vi "oax_gsTimebase Plot.vi"() -> ()   [LabVIEW 2017]
doc: "This is Order Analysis Toolkit demo VI."
uses:
  <vilib>/addons/Sound and Vibration/Order Analysis/Tach Process/SoundVib_TachProcess.lvlib
  <vilib>/addons/Sound and Vibration/Order Analysis/Resample Order Tracking/SoundVib_OrderTracking.lvlib
  <vilib>/Waveform/WDTOps.llb/WDT Waveform Duration DBL.vi
  <vilib>/addons/Sound and Vibration/Order Analysis/Data Presentation/SoundVib_MCMDisplay.lvlib
  <vilib>/addons/Sound and Vibration/Order Analysis/Data Presentation/SVX Orbit and Timebase Plot (Unfiltered).vi
  <vilib>/addons/Sound and Vibration/Order Analysis/Data Presentation/SubVIs/OAT MCM Channel Property.ctl
  <vilib>/addons/Sound and Vibration/Order Analysis/Data Presentation/SVX Orbit and Timebase Plot (Filtered) (N Ch - 1 Order).vi
  <vilib>/addons/_XControls/Timebase Plot/SVX Timebase.xctl
panel:
  in  "samples/rev wanted":i32=64
  in  "order to display":dbl=1.0 min=0.0 format="%.2f"
  in  "plot type":u16(ring) items=["unfiltered plot", "filtered plot"]
  in  "timebase plot display revolutions":cluster{"duration [rev]":dbl}={"duration [rev]"=8.0} {"duration [rev]" format="%.2f"}
  out "Timebase plot":T1(xcontrol) caption="Y axis"
  in  "STOP":bool
  in  "Select Data":i32(listbox)
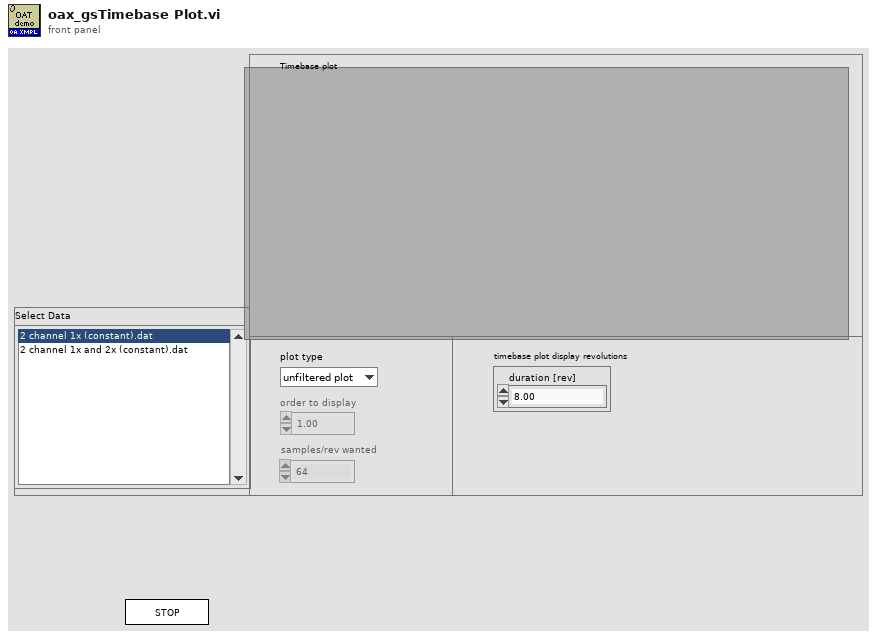
[diagram p1: front panel]
types:
  T1 = cluster{"X":dbl[], "Y":dbl[], "reference":dbl[], "plot type":enum16{"Filtered Plot", "Unfiltered Plot"}, "attribute":variant}[][]
  T2 = typedef "OAT MCM Channel Property.ctl" = cluster{"direction":u16, "probe angle [deg]":u16, "pair":u16}
  T3 = cluster{"unwrap phase? (T)":bool, "unit in degree? (F)":bool, "unwrap phase? (T) 2":bool}
  T4 = typedef "SoundVib_TachProcess.lvlib/speed profile.ctl" = cluster{"time [s]":dbl[], "speed [RPM]":dbl[]}
  T5 = typedef "svc_Resampled Channel Info.ctl" = cluster{"channel name":string, "description":string, " channel info":T6}
  T6 = typedef "svc_Channel Info.ctl" = cluster{"sensor sensitivity":dbl, "engineering units":T7, "dB reference":dbl, "custom label":string, "weighting filter":T8, "pregain":dbl}
  T7 = typedef "svc_Engineering Units Text Ring.ctl" = u16
  T8 = typedef "svc_Weighting Filter Text Ring.ctl" = u16
  T9 = typedef "OAT Position Info.ctl" = cluster{"positions [s]":dbl[], "samples/rev":dbl}
  T10 = cluster{"probe x":dbl[], "probe y":dbl[], "reference":dbl[], "plot type":enum16{"Filtered Plot", "Unfiltered Plot"}, "attribute":variant}[][]
  T11 = cluster{"time/rev/rpm":dbl[], "magnitude":dbl[]}[][]
  T12 = typedef "svc_Spectrum Info.ctl" = cluster{"channel name":string, "description":string, "x-axis units":T13, "spectral info":cluster{"spectrum type":T14, "linear/dB":enum16{"linear", "dB"}, "window":u16, "window size":i32, "FFT size":i32}, "engineering units":T7, "custom label":string, "dB reference [EU]":dbl, "peak units":enum16{"rms", "peak", "peak-peak"}, "weighting filter":T8, "spectral density?":bool, "unit label":string, "spectrum skewed?":bool, "complimentary spectrum units":T15}
  T13 = typedef "svc_X-Axis Units.ctl" = u16
  T14 = typedef "svc_Spectrum Type.ctl" = enum16{"FFT Spectrum [complex]", "Amplitude [Magnitude]", "Power [Magnitude^2]", "Cross Spectrum [complex]", "Frequency Response [Complex]"}
  T15 = typedef "svc_Complimentary Spectrum Units.ctl" = enum16{"none", "radians", "degrees", "cycles", "imaginary"}
  T16 = cluster{"time/rev/rpm":dbl[], "magnitude":dbl[]}[]
  T17 = cluster{"pulse / rev":i32, "threshold (auto)":dbl, "slope (Rising)":u16}
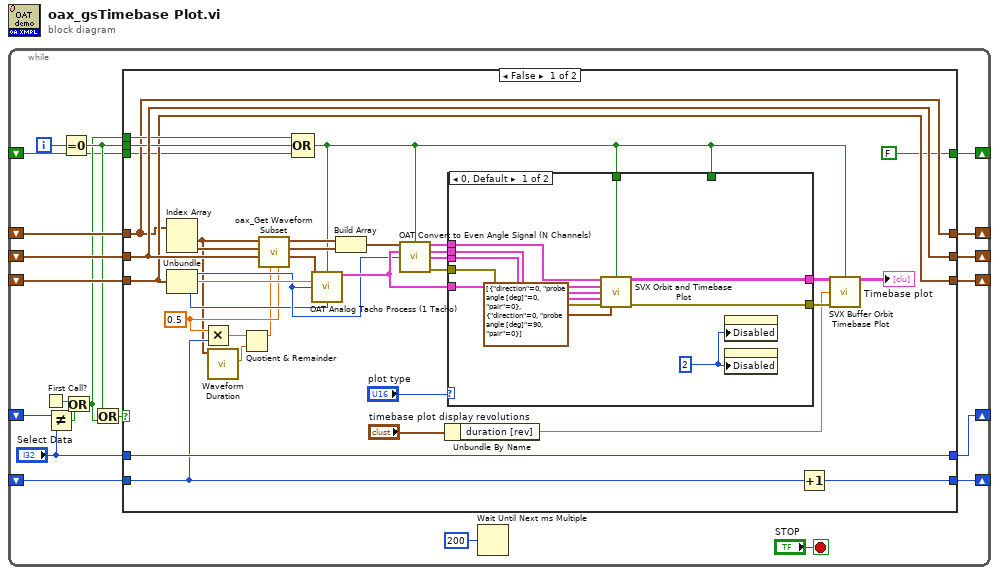
[diagram p0: block diagram]
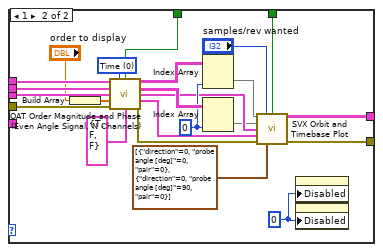
[diagram p2: hidden frame]
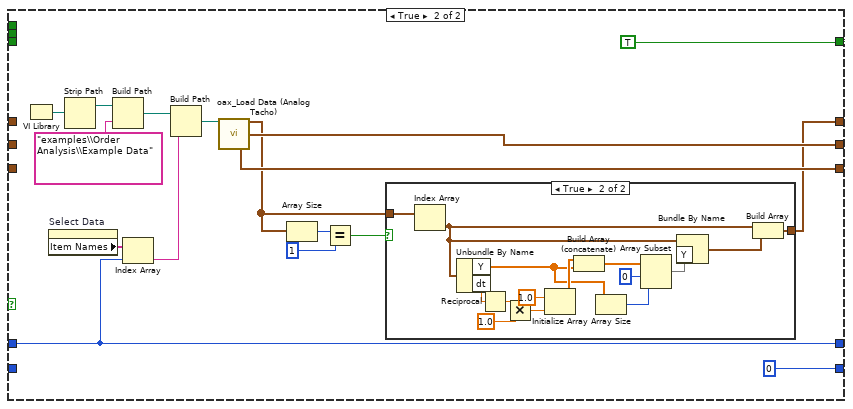
[diagram p3: hidden frame]
diagram:
  n1 = while {
    shift-right: [w17] -> _
    shift-left: _ -> [w18]
    shift-right: [w15] -> _
    shift-left: _ -> [w21]
    shift-right: [w14] -> _
    shift-left: _ -> [w19]
    shift-right: [w13] -> _
    shift-left: _ -> [w12]
    shift-right: [w3] -> _
    shift-left: _ -> [w4]
    shift-right: [w2] -> _
    shift-left: _ -> [w1]
    i -> [w11]
    stop <- "STOP" stop-if-true
    n2 = First Call?() -> (First Call?: T/F=w7:bool)
    n3 = Not Equal?(x=w18, y="Select Data") -> (x != y?=w6:bool)
    n4 = Equal To 0?(x=w11) -> (x = 0?=w10:bool)
    n5 = Or(x=w7, y=w6) -> (x .or. y?=w5:bool)
    n6 = Or(x=w10, y=w5) -> (x .or. y?=w9:bool)
    n7 = case shown="False" w9 {
      tunnel: w21 -> [w36 _]
      tunnel: w19 -> [w54 _]
      tunnel: [w55 w105] -> w17
      tunnel: "Select Data" -> [w55 w105]
      tunnel: [w36 w90] -> w15
      tunnel: [w54 w103] -> w14
      tunnel: [w47 w102] -> w13
      tunnel: w12 -> [w47 _]
      tunnel: w5 -> [w51 _]
      tunnel: w10 -> [w50 _]
      tunnel: w4 -> [w41 _]
      tunnel: [w43 0] -> w3
      tunnel: [FALSE TRUE] -> w2
      tunnel: w1 -> [w35 _]
      frame False {
        w42 = 0.5 ("y")
        n8 = Index Array(array=w36) -> (element #1=w40:waveform(dbl), element #2=w48:waveform(dbl))  [unwired: 2 in]
        n9 = Unbundle(w47) -> ("pulse / rev"=w45:i32, "threshold (auto)"=w46:dbl, "slope (Rising)"=w44:u16)
        n10 = Multiply(x=w42, y=w41) -> (x*y=w38:dbl)
        n11 = call-poly <vilib>:"Waveform Duration.vi"("waveform in"=w40) -> ("duration"=w39:dbl)  [unwired: 8 in, 2 out]
        n12 = Quotient & Remainder(x=w38, y=w39) -> (x-y*floor(x/y)=w37:dbl)  [unwired: 1 out]
        n13 = call <vilib>:"oax_Get Waveform Subset.vi"("duration"=w42, "start index"=w37, "Tach Signal"=w54, "Vibration Signal Y"=w48, "Vibration Signal X"=w40) -> ("Tach Signal out"=w52:waveform(dbl), "Vibration Signal Y out"=w53:waveform(dbl), "Vibration Signal X out"=w49:waveform(dbl))  [unwired: 3 in, 1 out]
        n14 = Compound Arithmetic op=OR(w51, w50, w35) -> (w26:bool)
        n15 = call <vilib>:"OAT Analog Tacho Process (1 Tacho).vi"("analog tacho signal"=w52, "reset? (F)"=w26, "threshold (auto)"=w46, "pulse/revolution (1)"=w45, "slope (Rising)"=w44) -> ("speed profile"=w56:T4)  [unwired: 6 in, 4 out]
        n16 = Build Array(w49, w53) -> (w33:waveform(dbl)[])
        n17 = call <vilib>:"OAT Convert to Even Angle Signal (N Channels).vi"("scaled signals [EU]"=w33, "reset? (F)"=w26, "speed profile"=w56, "pulse/revolution (1)"=w45) -> ("even-angle signals"=w32:cluster{"r0":dbl, "dr":dbl, "Y":dbl[]}[], "even-angle channel info"=w30:T5[], "even-angle position info"=w31:T9, "error out"=w29:errorcluster)  [unwired: 7 in, 1 out]
        n18 = Unbundle By Name("timebase plot display revolutions") -> ("duration [rev]"=w22:dbl)
        n19 = case shown="0, Default" "plot type" {
          tunnel: w32 -> [w61 w89]
          tunnel: w56 -> [w65 _]
          tunnel: w31 -> [w64 w87]
          tunnel: [w66 w68] -> w27
          tunnel: w30 -> [w60 w88]
          tunnel: w29 -> [w59 w86]
          tunnel: w26 -> [w63 w83]
          tunnel: w26 -> [_ w77]
          tunnel: [w57 w67] -> w24
          frame 0, Default {
            w62 = u8 2 ("Disabled")
            n20 = call-poly <vilib>:"SVX Orbit and Timebase Plot.vi"("even-angle signals"=w61, "reset? (F)"=w63, "even-angle channel info"=w60, "even-angle position info"=w64, "speed profile"=w65, "error in (no error)"=w59, "channel properties"=T2[] [{"direction"=0, "probe angle [deg]"=0, "pair"=0}, {"direction"=0, "probe angle [deg]"=90, "pair"=0}]) -> ("orbit/timebase plot"=w66:T10, "error out"=w57:errorcluster)  [unwired: 5 in, 2 out]
            n21 = property on="order to display" class="DigNum (strict)"("Disabled"=w62) -> ()  [unwired: 2 in, 2 out]
            n22 = property on="samples/rev wanted" class="DigNum (strict)"("Disabled"=w62) -> ()  [unwired: 2 in, 2 out]
          }
          frame 1 {
            w78 = u8 0 ("Disabled")
            w79 = u16 0 items=["Time", "Revolution", "RPM"] ("X axis selection")
            w80 = 0 ("disabled index (col)")
            n23 = Build Array("order to display") -> (w82:dbl[])
            n24 = call <vilib>:"OAT Order Magnitude and Phase (Even Angle Signal, N Channels).vi"("even-angle signals"=w89, "x-axis selection"=w79, "reset? (F)"=w83, "even-angle channel info"=w88, "even-angle position info"=w87, "orders to compute (1.0)"=w82, "error in (no error)"=w86, "view"=T3 {"unwrap phase? (T)"=TRUE, "unit in degree? (F)"=FALSE, "unwrap phase? (T) 2"=FALSE} ("phase setting")) -> ("magnitudes [RMS]"=w85:T11, "phases [phase lag]"=w84:cluster{"time/rev/rpm":dbl[], "phase":dbl[]}[][], "magnitude/phase position info"=w73:T9, "magnitudes info"=w70:T12[], "error out"=w81:errorcluster)  [unwired: 2 in, 1 out]
            n25 = Index Array(array=w85, index (col)=w80) -> (element=w74:T16)  [unwired: 1 in]
            n26 = Index Array(array=w84, index (col)=w80) -> (element=w72:cluster{"time/rev/rpm":dbl[], "phase":dbl[]}[])  [unwired: 1 in]
            n27 = call-poly <vilib>:"SVX Orbit and Timebase Plot.vi"("magnitudes [RMS]"=w74, "samples/rev wanted"="samples/rev wanted", "reset? (F)"=w77, "phases [phase lag]"=w72, "magnitude/phase position info"=w73, "magnitudes info"=w70, "error in (no error)"=w81, "channel properties"=T2[] [{"direction"=0, "probe angle [deg]"=0, "pair"=0}, {"direction"=0, "probe angle [deg]"=90, "pair"=0}]) -> ("orbit/timebase plot"=w68:T10, "error out"=w67:errorcluster)  [unwired: 4 in, 2 out]
            n28 = property on="order to display" class="DigNum (strict)"("Disabled"=w78) -> ()  [unwired: 2 in, 2 out]
            n29 = property on="samples/rev wanted" class="DigNum (strict)"("Disabled"=w78) -> ()  [unwired: 2 in, 2 out]
          }
        }
        n30 = Increment(x=w41) -> (x+1=w43:i32)
        n31 = call <vilib>:"SVX Buffer Orbit Timebase Plot.vi"("orbit/timebase plot in"=w27, "reset? (F)"=w26, "buffer size (rev)"=w22, "error in (no error)"=w24) -> ("orbit/timebase plot out"=→"Timebase plot":T10)  [unwired: 10 in, 1 out]
      }
      frame True {
        n32 = VI Library() -> (path=w98:path)
        n33 = property on="Select Data" class="LstBox (strict)"() -> ("Item Names"=w106:string[])  [unwired: 2 in, 2 out]
        n34 = Strip Path(path=w98) -> (stripped path=w97:path)  [unwired: 1 out]
        n35 = Build Path(base path=w97, name or relative path="examples\\Order Analysis\\Example Data") -> (appended path=w101:path)
        n36 = Index Array(array=w106, index=w105) -> (element=w100:string)
        n37 = Build Path(base path=w101, name or relative path=w100) -> (appended path=w99:path)
        n38 = call <vilib>:"oax_Load Data (Analog Tacho).vi"("Data Path In"=w99) -> ("vibration data"=w91:waveform(dbl)[], "analog tacho signal"=w103:waveform(dbl), "tacho info"=w102:T17)  [unwired: 8 in, 4 out]
        n39 = Array Size(array=w91) -> (size(s)=w94:i32)
        n40 = Equal?(x=w94, y=1) -> (x = y?=w92:bool)
        n41 = case shown="True" w92 {
          tunnel: w91 -> [w107 w122]
          tunnel: [w107 w121] -> w90
          frame False {
          }
          frame True {
            n42 = Index Array(array=w122) -> (element=w120:waveform(dbl))  [unwired: 1 in]
            n43 = Unbundle By Name(w120) -> ("Y"=w109:dbl[], "dt"=w118:dbl)
            n44 = Reciprocal(x=w118) -> (1/x=w117:dbl)
            n45 = Multiply(x=w117, y=1.0) -> (x*y=w115:dbl)
            n46 = Initialize Array(1.0 ("element"), w115) -> (w111:dbl[])
            n47 = Build Array (concatenate)(w111, w109) -> (w113:dbl[])
            n48 = Array Size(array=w109) -> (size(s)=w110:i32)
            n49 = Array Subset(array=w113, index=0, length=w110) -> (w108:dbl[])
            n50 = Bundle By Name(cluster=w120, "Y"=w108) -> (w119:waveform(dbl))
            n51 = Build Array(w120, w119) -> (w121:waveform(dbl)[])
          }
        }
      }
    }
    n52 = Wait Until Next ms Multiple(millisecond multiple=u32 200) -> ()  [unwired: 1 out]
  }
